vi "Write File Tree.vi"(8 "error in (no error)":errorcluster, 10 "File Tree Reference":refnum<vi>, 11 "File Tree In":refnum<class "File Tree.lvclass">) -> (0 "error out":errorcluster, 3 "File Tree Out":refnum<class "File Tree.lvclass">)   [LabVIEW 2020, in "File Tree.lvclass"]
uses:
  File Tree.lvclass
  File Tree.lvclass/File Tree.ctl
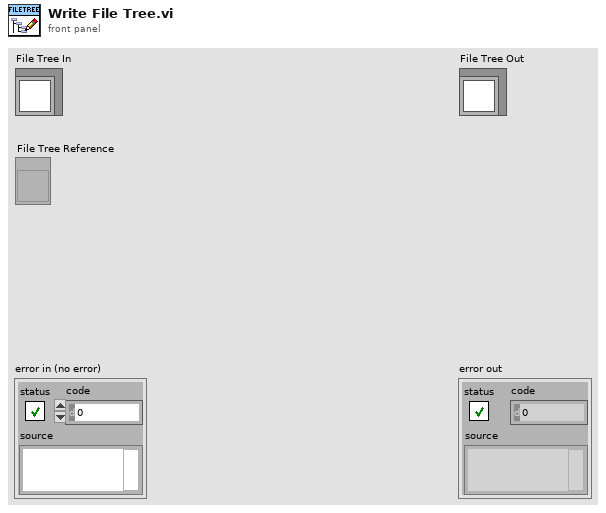
[diagram p1: front panel]
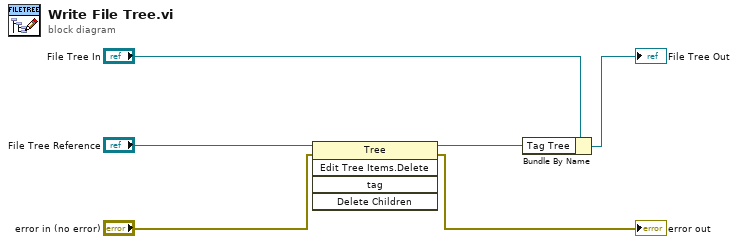
[diagram p0: block diagram]
diagram:
  n1 = invoke class="Tree" method="Edit Tree Items.Delete"(reference="File Tree Reference", error in="error in (no error)") -> (reference out=w3:refnum<vi>, error out=→"error out":errorcluster)  [unwired: 3 in, 3 out]
  n2 = Bundle By Name(cluster="File Tree In", "Tag Tree"=w3) -> (→"File Tree Out":refnum<class "File Tree.lvclass">)
